vi "ExcelBinData.vi"(5 "step":string, 6 "start row":i32, 7 "jobno":string, 8 "error in (no error) 2":errorcluster, 9 "report in":refnum<class "NI_report.lvclass">, 10 "error in (no error)":errorcluster, 11 "connection reference 2":T1) -> (0 "error out 2":errorcluster, 1 "report out":refnum<class "NI_report.lvclass">, 2 "error out":errorcluster, 3 "connection reference":T1)   [LabVIEW 2012]
uses:
  <vilib>/addons/database/Connection.llb/Conn ObjectReference.ctl
  <vilib>/Utility/NIReport.llb/NI_report.lvclass
  <vilib>/addons/database/Auxilliary.llb/DB Tools Cursor Type.ctl
  <vilib>/addons/database/Connection.llb/Conn Execute.vi
  <vilib>/addons/database/Recordset.llb/Rec Fetch String Data (R).vi
  <vilib>/addons/database/Recordset.llb/Rec Fetch Integer Data (R).vi
  <vilib>/addons/database/Recordset.llb/Rec Destroy - Connection.vi
  <vilib>/addons/database/NI_Database_API.lvlib
  <vilib>/Utility/NIReport.llb/Excel/NI_Excel.lvclass
panel:
  out "x .and. y?":bool
  out "substring":string
  in  "start (0, 0)":cluster{"start row":i32, "start column":i32}
  out "concatenated string":string
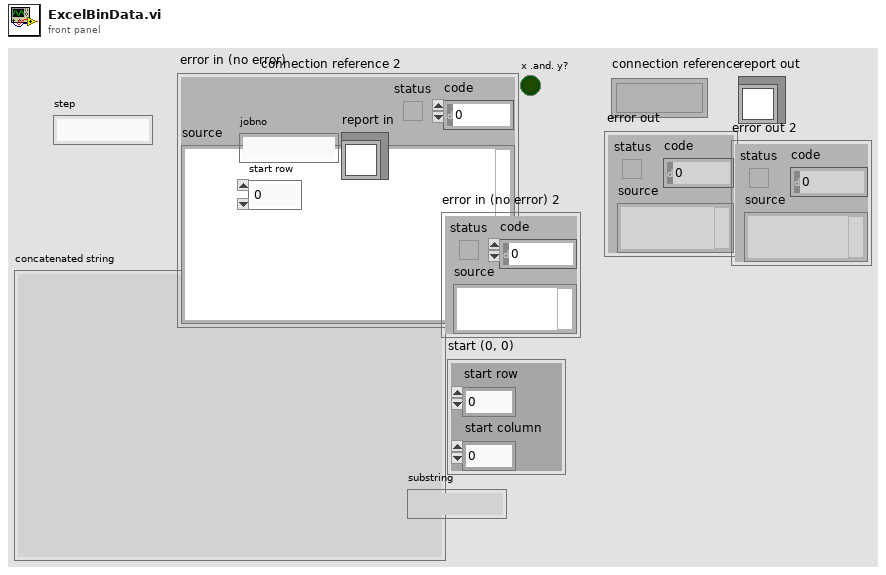
[diagram p1: front panel]
types:
  T1 = typedef "NI_Database_API.lvlib/Conn ObjectReference.ctl" = refnum<k1>
  T2 = typedef "NI_Database_API.lvlib/DB Tools Cursor Type.ctl" = enum16{"forward-only", "keyset", "dynamic", "static"}
  T3 = typedef "NI_Database_API.lvlib/Rec ObjectReference.ctl" = refnum<k1>
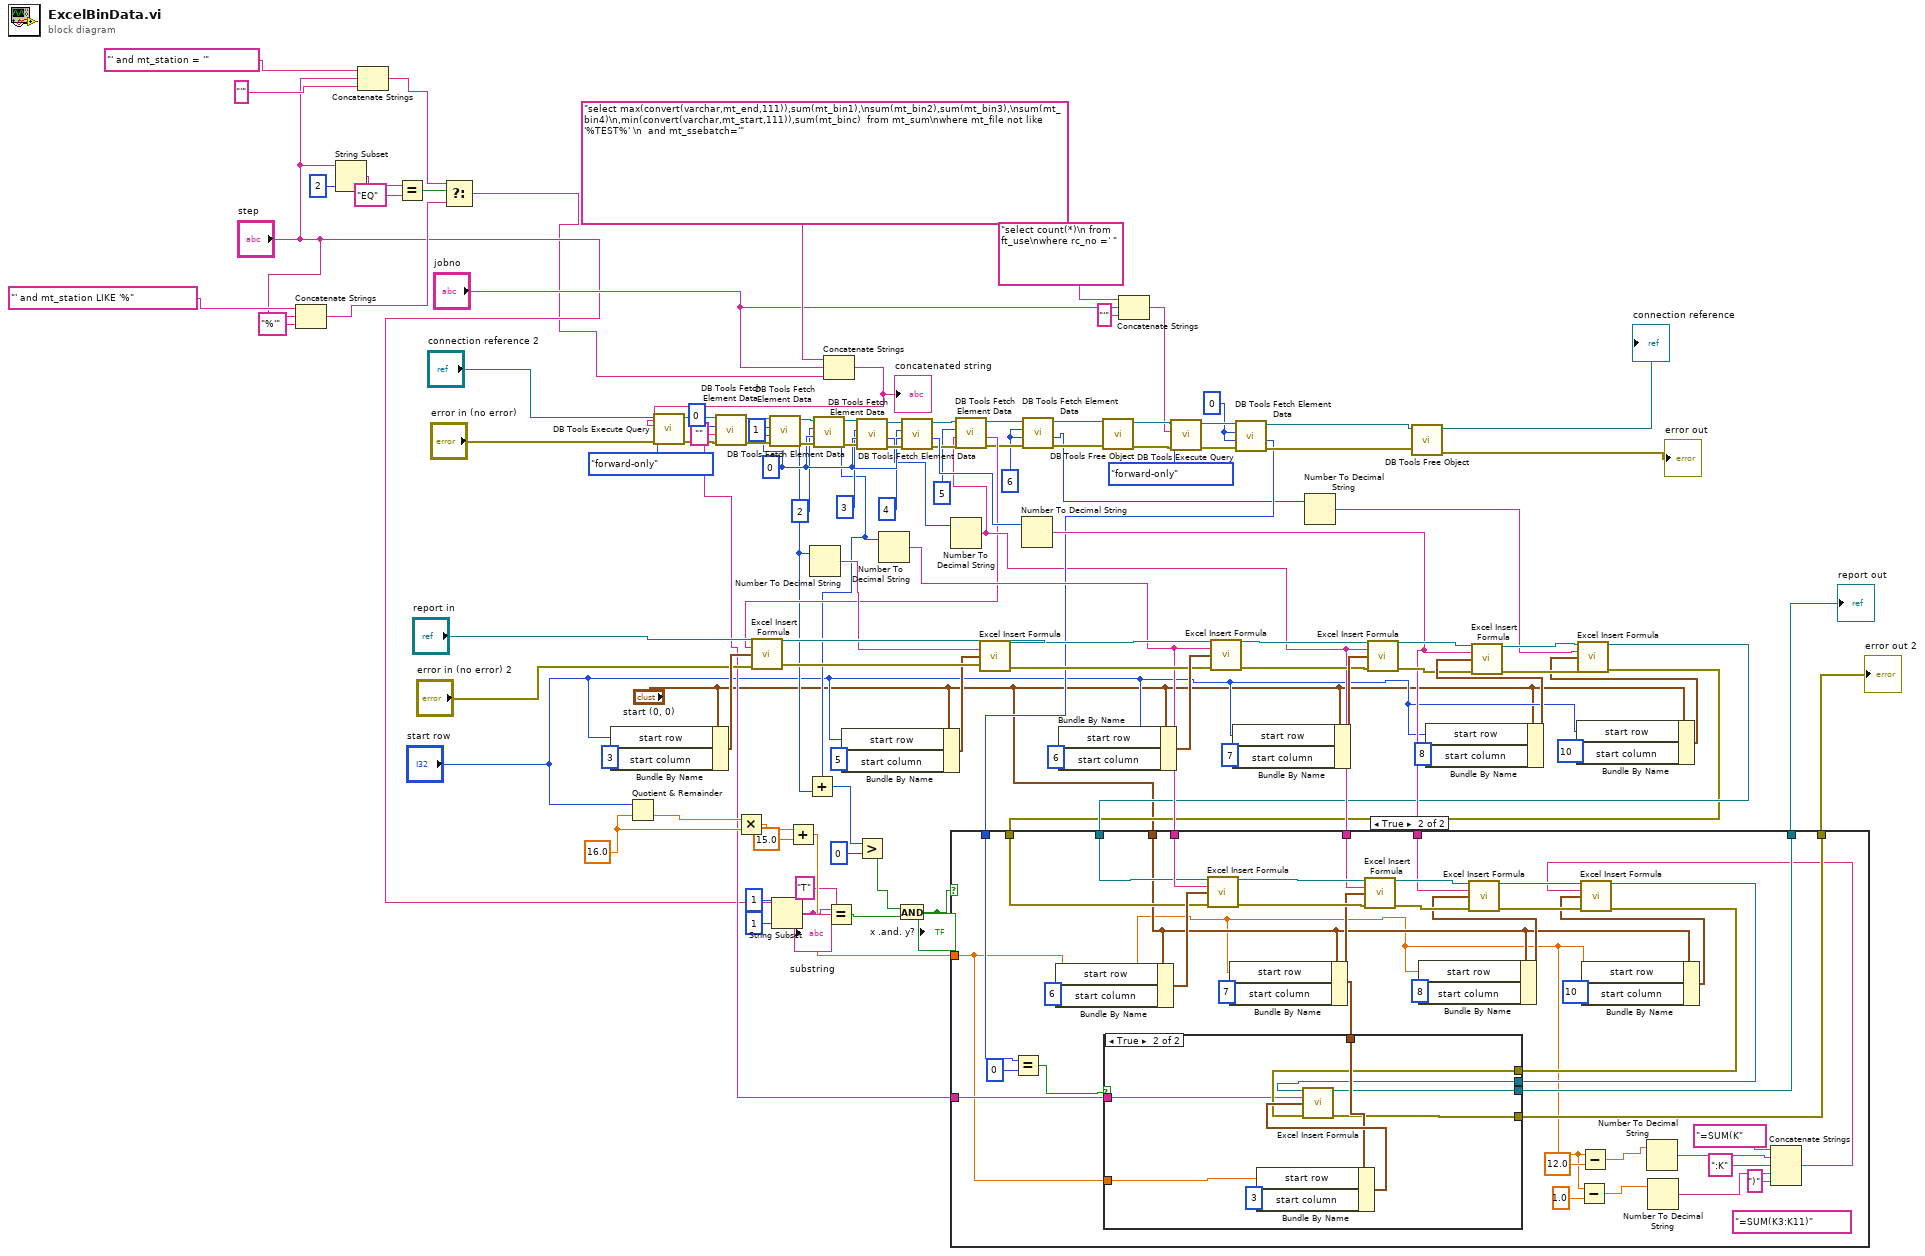
[diagram p0: block diagram]
diagram:
  w30 = 6
  w45 = 0
  w67 = 16.0 ("y")
  w98 = 0
  n1 = Concatenate Strings("' and mt_station LIKE '%" ("string"), "step", "%'" ("string")) -> (w6:string)
  n2 = String Subset(string="step", length (rest)=2 ("length (rest)")) -> (substring=w11:string)  [unwired: 1 in]
  n3 = Concatenate Strings("' and mt_station = '" ("string"), "step", "'" ("string")) -> (w2:string)
  n4 = Equal?(x=w11, y="EQ") -> (x = y?=w7:bool)
  n5 = Select(t=w2, s=w7, f=w6) -> (s? t:f=w1:string)
  n6 = Bundle By Name(cluster="start (0, 0)", "start row"="start row", "start column"=3) -> (w93:cluster{"start row":i32, "start column":i32})
  n7 = Quotient & Remainder(x="start row", y=w67) -> (floor(x/y)=w68:dbl)  [unwired: 1 out]
  n8 = Multiply(x=w68, y=w67) -> (x*y=w66:dbl)
  n9 = String Subset(string="step", offset (0)=1, length (rest)=1 ("length (rest)")) -> (substring=w18:string)
  "substring" <- w18
  n10 = Add(x=w66, y=15.0) -> (x+y=w61:dbl)
  n11 = Concatenate Strings("select max(convert(varchar,mt_end,111)),sum(mt_bin1),\nsum(mt_bin2),sum(mt_bin3),\nsum(mt_bin4)\n,min(convert(varchar,mt_start,111)),sum(mt_binc)  from mt_sum\nwhere mt_file not like '%TEST%' \n  and mt_ssebatch='", "jobno", w1) -> (w112:string)
  "concatenated string" <- w112
  n12 = call-poly <vilib>:"DB Tools Execute Query.vi"("error in (no error)"="error in (no error)", "cursor type"=DB_Tools_Cursor_Type."forward-only", "SQL query"=w112, "connection reference"="connection reference 2") -> ("error out"=w109:errorcluster, "recordset reference"=w110:T3)  [unwired: 4 in]
  n13 = call-poly <vilib>:"DB Tools Fetch Element Data.vi"("error in (no error)"=w109, "type"="", "column index"=0, "recordset reference"=w110) -> ("error out"=w105:errorcluster, "data"=w43:string, "recordset reference out"=w106:T3)  [unwired: 3 in]
  n14 = call-poly <vilib>:"DB Tools Fetch Element Data.vi"("error in (no error)"=w105, "type"=w98, "column index"=1, "recordset reference"=w106) -> ("error out"=w101:errorcluster, "data"=w36:i32, "recordset reference out"=w104:T3)  [unwired: 3 in]
  n15 = Number To Decimal String(number=w36) -> (decimal integer string=w88:string)  [unwired: 1 in]
  n16 = call-poly <vilib>:"DB Tools Fetch Element Data.vi"("error in (no error)"=w101, "type"=w98, "column index"=2, "recordset reference"=w104) -> ("error out"=w100:errorcluster, "data"=w35:i32, "recordset reference out"=w103:T3)  [unwired: 3 in]
  n17 = Add(x=w35, y=w36) -> (x+y=w37:i32)
  n18 = Equal?(x=w18, y="T") -> (x = y?=w15:bool)
  n19 = Bundle By Name(cluster="start (0, 0)", "start row"="start row", "start column"=5) -> (w87:cluster{"start row":i32, "start column":i32})
  n20 = call-poly <vilib>:"DB Tools Fetch Element Data.vi"("error in (no error)"=w100, "type"=w98, "column index"=3, "recordset reference"=w103) -> ("error out"=w99:errorcluster, "data"=w82:i32, "recordset reference out"=w102:T3)  [unwired: 3 in]
  n21 = Greater?(x=w37, y=0) -> (0:w16:bool)
  n22 = Number To Decimal String(number=w35) -> (decimal integer string=w62:string)  [unwired: 1 in]
  n23 = And(x=w16, y=w15) -> (x .and. y?=w14:bool)
  "x .and. y?" <- w14
  n24 = call-poly <vilib>:"DB Tools Fetch Element Data.vi"("error in (no error)"=w99, "type"=w98, "column index"=4, "recordset reference"=w102) -> ("error out"=w41:errorcluster, "data"=w81:i32, "recordset reference out"=w42:T3)  [unwired: 3 in]
  n25 = Number To Decimal String(number=w82) -> (decimal integer string=w39:string)  [unwired: 1 in]
  n26 = call-poly <vilib>:"DB Tools Fetch Element Data.vi"("error in (no error)"=w41, "type"=w39, "column index"=5, "recordset reference"=w42) -> ("error out"=w32:errorcluster, "data"=w38:string, "recordset reference out"=w34:T3)  [unwired: 3 in]
  n27 = call <vilib>:"Excel Insert Formula.vi"("report in"="report in", "formula"=w38, "start (0, 0)"=w93, "error in (no error)"="error in (no error) 2") -> ("report out"=w91:refnum<class "NI_report.lvclass">, "error out"=w90:errorcluster)  [unwired: 10 in]
  n28 = call <vilib>:"Excel Insert Formula.vi"("report in"=w91, "formula"=w88, "start (0, 0)"=w87, "error in (no error)"=w90) -> ("report out"=w83:refnum<class "NI_report.lvclass">, "error out"=w85:errorcluster)  [unwired: 10 in]
  n29 = Number To Decimal String(number=w81) -> (decimal integer string=w63:string)  [unwired: 1 in]
  n30 = call-poly <vilib>:"DB Tools Fetch Element Data.vi"("error in (no error)"=w32, "type"=w30, "column index"=w30, "recordset reference"=w34) -> ("error out"=w31:errorcluster, "data"=w29:i32, "recordset reference out"=w33:T3)  [unwired: 3 in]
  n31 = Bundle By Name(cluster="start (0, 0)", "start row"="start row", "start column"=6) -> (w86:cluster{"start row":i32, "start column":i32})
  n32 = call-poly <vilib>:"DB Tools Free Object.vi"("error in (no error)"=w31, "recordset reference"=w33) -> ("error out"=w57:errorcluster, "connection reference"=w58:T1)  [unwired: 8 in]
  n33 = Concatenate Strings("select count(*)\n from ft_use\nwhere rc_no =' " ("string"), "jobno", "'" ("string")) -> (w46:string)
  n34 = call-poly <vilib>:"DB Tools Execute Query.vi"("error in (no error)"=w57, "cursor type"=DB_Tools_Cursor_Type."forward-only", "SQL query"=w46, "connection reference"=w58) -> ("error out"=w55:errorcluster, "recordset reference"=w56:T3)  [unwired: 4 in]
  n35 = call <vilib>:"Excel Insert Formula.vi"("report in"=w83, "formula"=w62, "start (0, 0)"=w86, "error in (no error)"=w85) -> ("report out"=w76:refnum<class "NI_report.lvclass">, "error out"=w74:errorcluster)  [unwired: 10 in]
  n36 = Bundle By Name(cluster="start (0, 0)", "start row"="start row", "start column"=7) -> (w78:cluster{"start row":i32, "start column":i32})
  n37 = call-poly <vilib>:"DB Tools Fetch Element Data.vi"("error in (no error)"=w55, "type"=w45, "column index"=w45, "recordset reference"=w56) -> ("error out"=w53:errorcluster, "data"=w44:i32, "recordset reference out"=w54:T3)  [unwired: 3 in]
  n38 = Number To Decimal String(number=w29) -> (decimal integer string=w24:string)  [unwired: 1 in]
  n39 = call <vilib>:"Excel Insert Formula.vi"("report in"=w76, "formula"=w39, "start (0, 0)"=w78, "error in (no error)"=w74) -> ("report out"=w75:refnum<class "NI_report.lvclass">, "error out"=w73:errorcluster)  [unwired: 10 in]
  n40 = call-poly <vilib>:"DB Tools Free Object.vi"("error in (no error)"=w53, "recordset reference"=w54) -> ("error out"=→"error out":errorcluster, "connection reference"=→"connection reference":T1)  [unwired: 8 in]
  n41 = Bundle By Name(cluster="start (0, 0)", "start row"="start row", "start column"=8) -> (w77:cluster{"start row":i32, "start column":i32})
  n42 = call <vilib>:"Excel Insert Formula.vi"("report in"=w75, "formula"=w63, "start (0, 0)"=w77, "error in (no error)"=w73) -> ("report out"=w28:refnum<class "NI_report.lvclass">, "error out"=w27:errorcluster)  [unwired: 10 in]
  n43 = Bundle By Name(cluster="start (0, 0)", "start row"="start row", "start column"=10) -> (w20:cluster{"start row":i32, "start column":i32})
  n44 = call <vilib>:"Excel Insert Formula.vi"("report in"=w28, "formula"=w24, "start (0, 0)"=w20, "error in (no error)"=w27) -> ("report out"=w26:refnum<class "NI_report.lvclass">, "error out"=w25:errorcluster)  [unwired: 10 in]
  n45 = case shown="True" w14 {
    tunnel: "start (0, 0)" -> [_ w129]
    tunnel: w63 -> [_ w146]
    tunnel: w39 -> [_ w145]
    tunnel: w62 -> [_ w144]
    tunnel: w61 -> [_ w124]
    tunnel: [w114 w135] -> w60
    tunnel: [w115 w136] -> w59
    tunnel: w25 -> [w115 w142]
    tunnel: w26 -> [w114 w141]
    tunnel: w44 -> [_ w140]
    tunnel: w43 -> [_ w134]
    frame False {
    }
    frame True {
      (unwired) "=SUM(K3:K11)"
      n46 = Equal?(x=w140, y=0) -> (x = y?=w138:bool)
      n47 = Bundle By Name(cluster=w129, "start row"=w124, "start column"=6) -> (w154:cluster{"start row":i32, "start column":i32})
      n48 = call <vilib>:"Excel Insert Formula.vi"("report in"=w141, "formula"=w144, "start (0, 0)"=w154, "error in (no error)"=w142) -> ("report out"=w150:refnum<class "NI_report.lvclass">, "error out"=w148:errorcluster)  [unwired: 10 in]
      n49 = Bundle By Name(cluster=w129, "start row"=w124, "start column"=7) -> (w137:cluster{"start row":i32, "start column":i32})
      n50 = call <vilib>:"Excel Insert Formula.vi"("report in"=w150, "formula"=w145, "start (0, 0)"=w137, "error in (no error)"=w148) -> ("report out"=w149:refnum<class "NI_report.lvclass">, "error out"=w147:errorcluster)  [unwired: 10 in]
      n51 = Bundle By Name(cluster=w129, "start row"=w124, "start column"=8) -> (w143:cluster{"start row":i32, "start column":i32})
      n52 = call <vilib>:"Excel Insert Formula.vi"("report in"=w149, "formula"=w146, "start (0, 0)"=w143, "error in (no error)"=w147) -> ("report out"=w133:refnum<class "NI_report.lvclass">, "error out"=w132:errorcluster)  [unwired: 10 in]
      n53 = Subtract(x=w124, y=1.0) -> (x-y=w119:dbl)
      n54 = Subtract(x=w124, y=12.0) -> (x-y=w122:dbl)
      n55 = Bundle By Name(cluster=w129, "start row"=w124, "start column"=10) -> (w127:cluster{"start row":i32, "start column":i32})
      n56 = Number To Decimal String(number=w122) -> (decimal integer string=w121:string)  [unwired: 1 in]
      n57 = Number To Decimal String(number=w119) -> (decimal integer string=w118:string)  [unwired: 1 in]
      n58 = Concatenate Strings("=SUM(K" ("string"), w121, ":K" ("string"), w118, ")" ("string")) -> (w116:string)
      n59 = call <vilib>:"Excel Insert Formula.vi"("report in"=w133, "formula"=w116, "start (0, 0)"=w127, "error in (no error)"=w132) -> ("report out"=w131:refnum<class "NI_report.lvclass">, "error out"=w130:errorcluster)  [unwired: 10 in]
      n60 = case shown="True" w138 {
        tunnel: w124 -> [_ w163]
        tunnel: w137 -> [_ w162]
        tunnel: w130 -> [w155 w161]
        tunnel: [w155 w160] -> w136
        tunnel: w131 -> [w156 w159]
        tunnel: [w156 w158] -> w135
        tunnel: w134 -> [_ w157]
        frame False {
        }
        frame True {
          n61 = Bundle By Name(cluster=w162, "start row"=w163, "start column"=3) -> (w164:cluster{"start row":i32, "start column":i32})
          n62 = call <vilib>:"Excel Insert Formula.vi"("report in"=w159, "formula"=w157, "start (0, 0)"=w164, "error in (no error)"=w161) -> ("report out"=w158:refnum<class "NI_report.lvclass">, "error out"=w160:errorcluster)  [unwired: 10 in]
        }
      }
    }
  }
  "report out" <- w60
  "error out 2" <- w59
